vi "Read I32.vi"(7 "key":string, 8 "error in (no error)":errorcluster, 9 "default value":i32, 11 "Configuration In":refnum<class "Mock Configuration.lvclass">) -> (0 "error out":errorcluster, 1 "value":i32, 3 "Configuration Out":refnum<class "Mock Configuration.lvclass">)   [LabVIEW 2020, in "Mock Configuration.lvclass"]
doc: "High-level function for reading configuration file data from process class. If the specified key is not present, it is added with the configured default value."
uses:
  Mock Configuration.lvclass
  C:/Program Files (x86)/National Instruments/LabVIEW 2020/vi.lib/Astemes/LMock/Mock.lvclass
  <vilib>/Astemes/LMock/Mock.lvclass
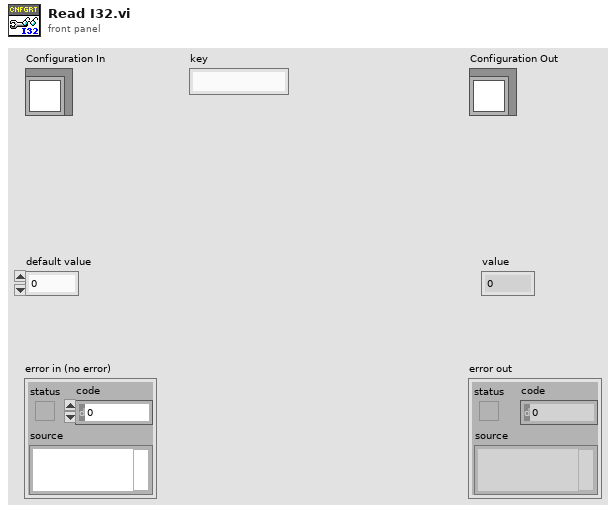
[diagram p1: front panel]
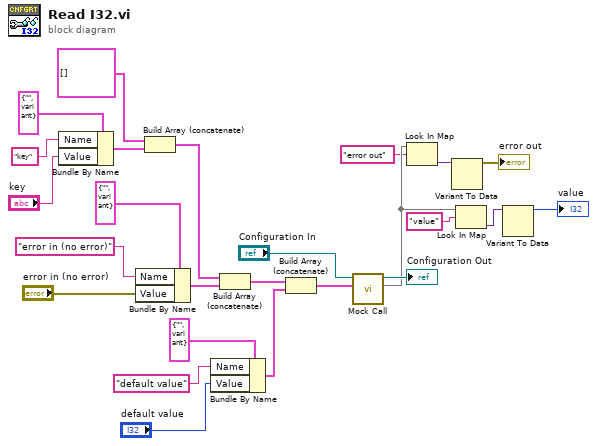
[diagram p0: block diagram]
diagram:
  n1 = Bundle By Name(cluster=cluster{"Name":string, "Value":variant} {"Name"="", "Value"=variant} ("element"), "Name"="key", "Value"="key") -> (w5:cluster{"Name":string, "Value":variant})
  n2 = Bundle By Name(cluster=cluster{"Name":string, "Value":variant} {"Name"="", "Value"=variant} ("element"), "Name"="error in (no error)", "Value"="error in (no error)") -> (w3:cluster{"Name":string, "Value":variant})
  n3 = Build Array (concatenate)(cluster{"Name":string, "Value":variant}[] [] ("Control Values"), w5) -> (w17:cluster{"Name":string, "Value":variant}[])
  n4 = Bundle By Name(cluster=cluster{"Name":string, "Value":variant} {"Name"="", "Value"=variant} ("element"), "Name"="default value", "Value"="default value") -> (w1:cluster{"Name":string, "Value":variant})
  n5 = Build Array (concatenate)(w17, w3) -> (w19:cluster{"Name":string, "Value":variant}[])
  n6 = Build Array (concatenate)(w19, w1) -> (w22:cluster{"Name":string, "Value":variant}[])
  n7 = call <vilib>:"Mock Call.vi"("Control Values"=w22, "Mock In"="Configuration In") -> ("Return Values"=w14:map{string, variant}, "Mock Out"=→"Configuration Out":refnum<class "Mock Configuration.lvclass">)  [unwired: 8 in]
  n8 = Look In Map(map=w14, key="error out") -> (value=w12:variant)  [unwired: 1 in, 1 out]
  n9 = Variant To Data(Variant=w12) -> (data=→"error out":errorcluster)  [unwired: 2 in, 1 out]
  n10 = Look In Map(map=w14, key="value") -> (value=w9:variant)  [unwired: 1 in, 1 out]
  n11 = Variant To Data(Variant=w9) -> (data=→"value":i32)  [unwired: 2 in, 1 out]
